vi "LIA.GetMagnitude.vi"(8 "error in (no error)":errorcluster, 11 "LIA.Simulated in":refnum<class "LIA.Simulated.lvclass">) -> (0 "error out":errorcluster, 2 "Magnitude":dbl, 3 "LIA.Simulated out":refnum<class "LIA.Simulated.lvclass">)   [LabVIEW 2017, in "LIA.Simulated.lvclass"]
uses:
  LIA.Simulated.lvclass
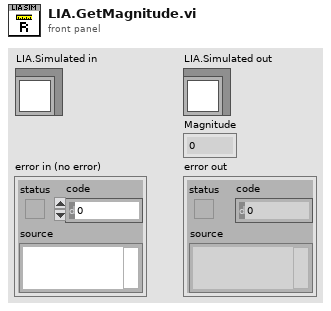
[diagram p1: front panel]
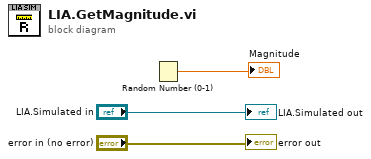
[diagram p0: block diagram]
diagram:
  n1 = Random Number (0-1)() -> (number: 0 to 1=→"Magnitude":dbl)
  "error out" <- "error in (no error)"
  "LIA.Simulated out" <- "LIA.Simulated in"
